vi "Choreo_DifferentialSample_GetChassisSpeeds.vi"(11 "ChoreoDifferentialSample":T2={"timestamp"=-999.0, "x"=0.0, "y"=0.0, "heading"=0.0, "velocityL"=0.0, "velocityR"=0.0, "angularVelocity"=0.0, "accelL"=0.0, "accelR"=0.0, "accelAngular"=0.0, "forceL"=0.0, "forceR"=0.0}) -> (3 "ChassisSpeeds":T1 {"vOmega" format="%10.3f"; "vY" format="%10.3f"; "vX" format="%10.3f"})   [LabVIEW 2019, in "ChoreoLib.lvlib"]
doc: "Returns the field-relative chassis speeds of this sample.\n\nInputs:\n -- ChoreoDifferentialSample - cluster - Differential sample.\n \nOutputs: \n -- ChassisSpeed - ChassisSpeed cluster - The field-relative chassis speeds of this sample."
uses:
  <vilib>/Rock Robotics/WPI/ThirdParty/JAS_Junk/TrajLib/TypeDef/CHASSIS_SPEEDS.ctl
  ChoreoLib.lvlib
  <vilib>/Rock Robotics/WPI/ThirdParty/JAS_Junk/TrajLib/Trajectory_Library.lvlib
  TypeDef/ChoreoDifferentialSample.ctl
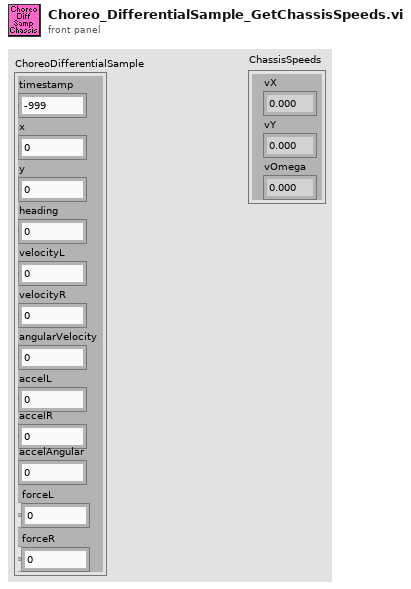
[diagram p1: front panel]
types:
  T1 = typedef "Trajectory_Library.lvlib/CHASSIS_SPEEDS.ctl" = cluster{"vX":dbl, "vY":dbl, "vOmega":dbl}
  T2 = typedef "ChoreoLib.lvlib/ChoreoDifferentialSample.ctl" = cluster{"timestamp":dbl, "x":dbl, "y":dbl, "heading":dbl, "velocityL":dbl, "velocityR":dbl, "angularVelocity":dbl, "accelL":dbl, "accelR":dbl, "accelAngular":dbl, "forceL":dbl, "forceR":dbl}
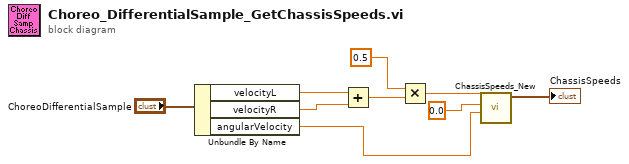
[diagram p0: block diagram]
diagram:
  n1 = Unbundle By Name("ChoreoDifferentialSample") -> ("velocityL"=w8:dbl, "velocityR"=w7:dbl, "angularVelocity"=w2:dbl)
  n2 = Add(x=w8, y=w7) -> (x+y=w6:dbl)
  n3 = Multiply(x=0.5, y=w6) -> (x*y=w4:dbl)
  n4 = call <vilib>:"ChassisSpeeds_New.vi"("vAngular"=w2, "vY"=0.0, "vX"=w4) -> ("CHASSIS"=→"ChassisSpeeds":T1)  [unwired: 8 in]
